vi "ZCAN_MsgDisplayBox.vi"(0 "帧类型":string, 2 "ID":u32, 5 "帧格式":string, 7 "Message Data":u8[](array[numeric]), 9 "data_len":u32) -> (6 "Output String":string)   [LabVIEW 2018]
doc: "用字符串显示解析（报文）。"
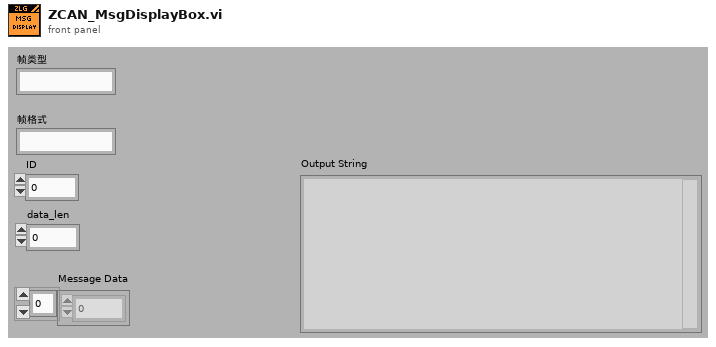
[diagram p1: front panel]
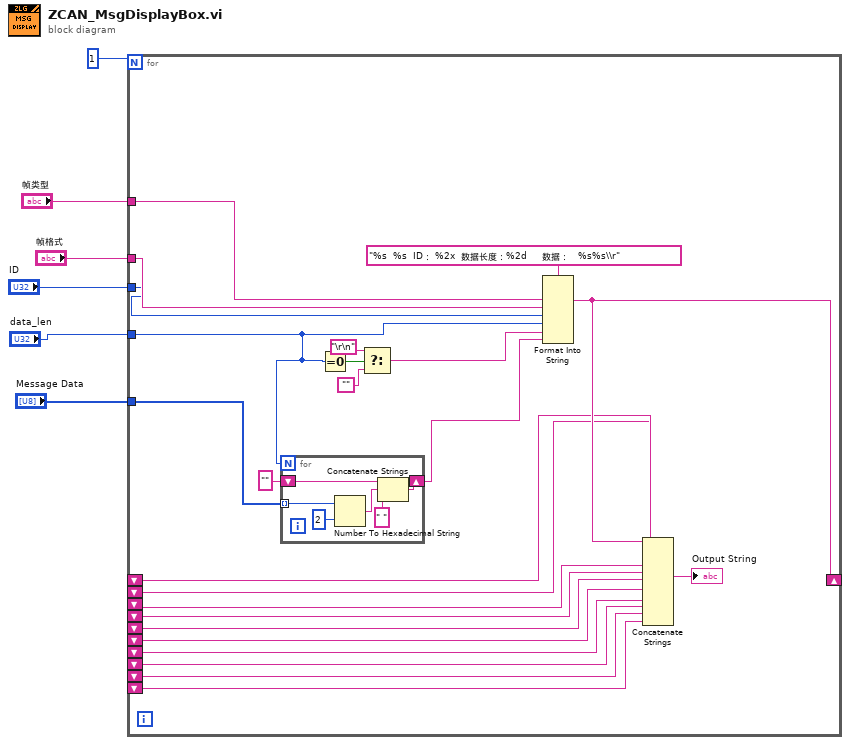
[diagram p0: block diagram]
diagram:
  n1 = for {
    N: 1 -> [_]
    shift-right: [w29] -> _
    shift-left: _ -> [w28]
    shift-left: _ -> [w27]
    shift-left: _ -> [w26]
    shift-left: _ -> [w25]
    shift-left: _ -> [w24]
    shift-left: _ -> [w23]
    shift-left: _ -> [w22]
    shift-left: _ -> [w21]
    shift-left: _ -> [w20]
    shift-left: _ -> [w19]
    tunnel: "ID" -> [w11]
    tunnel: "Message Data" -> [w8]
    tunnel: "帧格式" -> [w12]
    tunnel: "帧类型" -> [w13]
    tunnel: "data_len" -> [w7]
    n2 = for {
      N: w7 -> [_]
      shift-right: [w33] -> w9
      shift-left: "" -> [w31]
      tunnel: w8 -> [w32] mode=indexing
      n3 = Number To Hexadecimal String(1:i16 2 ("width (-)"), 2:w32) -> (0:w35:string)
      n4 = Concatenate Strings(w31, w35, " " ("string")) -> (w33:string)
    }
    n5 = Equal To 0?(x=w7) -> (x = 0?=w17:bool)
    n6 = Select(t="\r\n", s=w17, f="") -> (s? t:f=w14:string)
    n7 = Format Into String(format string="%s  %s  ID： %2x  数据长度：%2d     数据：   %s%s\\r", w13, w12, w11, w7, w14, w9) -> (resulting string=w29:string)  [unwired: 2 in, 1 out]
    n8 = Concatenate Strings(w29, w28, w27, w26, w25, w24, w23, w22, w21, w20, w19) -> (→"Output String":string)
  }
